vi "Copy_File.vi"(8 "error in (no error)":errorcluster, 9 "newName":string, 10 "sourcePath":path, 11 "AB_Dest_LLB in":refnum<class "AB_Dest_LLB.lvclass">) -> (0 "error out":errorcluster, 2 "destinationPath":path, 3 "AB_Dest_LLB out":refnum<class "AB_Dest_LLB.lvclass">)   [LabVIEW 2020, in "AB_Dest_LLB.lvclass"]
uses:
  <vilib>/AppBuilder/AB_Classes/Destination/Dest_LLB/AB_Dest_LLB.lvclass
  e:/builds/penguin/labview/branches/2020/dev/dist/vi.lib/AppBuilder/AB_Classes/Destination/AB_Destination.lvclass
  <resource>/Framework/Providers/Common/provcom_StringGlobals.vi
  <vilib>/AppBuilder/AB_Classes/Destination/AB_Destination.lvclass
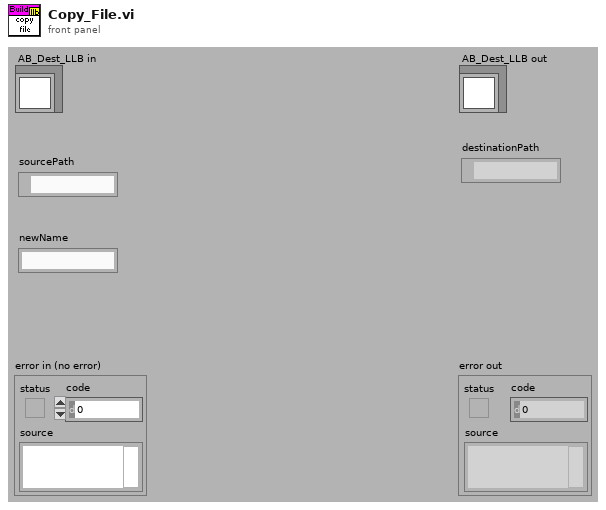
[diagram p1: front panel]
types:
  T1 = typedef "AB_Destination.ctl" = cluster{"destName":string, "path":path, "libraryName":string, "preserveHierarchy":bool, "eng_inBuild":bool, "eng_libraryReference":refnum<vi>, "eng_restictAddToNewLibrary":bool}
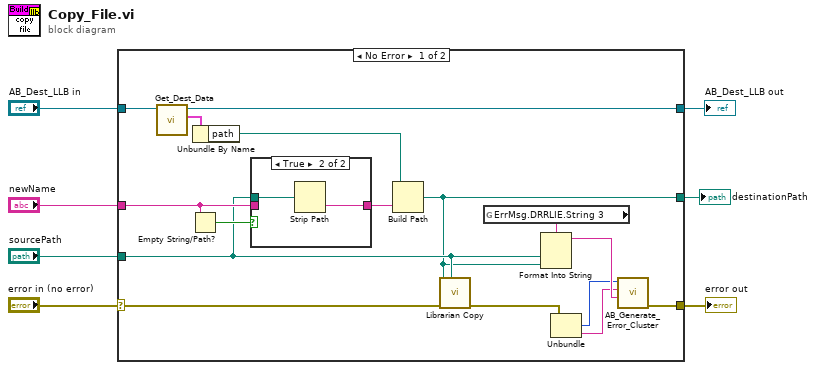
[diagram p0: block diagram]
diagram:
  n1 = case shown="No Error" "error in (no error)" {
    selector: "error in (no error)" -> [w20 w28]
    tunnel: [w12 w28] -> w2
    tunnel: [w16 w27] -> w6
    tunnel: "AB_Dest_LLB in" -> [w18 w27]
    tunnel: "sourcePath" -> [w10 _]
    tunnel: "newName" -> [w22 _]
    tunnel: [w9 _] -> w1
    frame No Error {
      n2 = call <vilib>:"Get_Dest_Data.vi"("Class in"=w18) -> ("destName"=w19:T1, "Class out"=w16:refnum<class "AB_Dest_LLB.lvclass">)  [unwired: 1 in, 8 out]
      n3 = Empty String/Path?(string/path=w22) -> (empty?=w23:bool)
      n4 = Unbundle By Name(w19) -> ("path"=w17:path)
      n5 = case shown="True" w23 {
        tunnel: [w24 w26] -> w21
        tunnel: w22 -> [w24 _]
        tunnel: w10 -> [_ w25]
        frame False {
        }
        frame True {
          n6 = Strip Path(path=w25) -> (name=w26:string)  [unwired: 1 out]
        }
      }
      n7 = Build Path(base path=w17, name or relative path=w21) -> (appended path=w9:path)
      n8 = call <vilib>:"Librarian Copy.vi"("source"=w10, "error in (no error)"=w20, "destination"=w9) -> ("error out"=w11:errorcluster)  [unwired: 2 in, 6 out]
      n9 = global read "provcom_StringGlobals.vi" "ErrMsg.DRRLIE.String 3"() -> (w8:string)
      n10 = Format Into String(format string=w8, w10, w9) -> (resulting string=w15:string)  [unwired: 2 in, 1 out]
      n11 = Unbundle(w11) -> ("code"=w14:i32, "source"=w13:string)  [unwired: 1 out]
      n12 = call <vilib>:"AB_Generate_Error_Cluster.vi"("Additional Message"=w15, "source"=w13, "Code"=w14) -> ("error out"=w12:errorcluster)  [unwired: 1 in, 7 out]
    }
    frame Error {
    }
  }
  "error out" <- w2
  "AB_Dest_LLB out" <- w6
  "destinationPath" <- w1
